vi "Inject.vi"(8 "error in (no error)":errorcluster, 9 "Injection Data":variant, 10 "Internal Message Queue":refnum<queue>, 11 "InteractionProcessor in":refnum<class "InteractionProcessor.lvclass">) -> (0 "error out":errorcluster, 3 "InteractionProcessor out":refnum<class "InteractionProcessor.lvclass">)   [LabVIEW 2023, in "HAF.lvlib" / "InteractionProcessor.lvclass"]
doc: "Add the Command Directors passed in the Message Data to the current set of Command Directors for processing."
uses:
  InteractionProcessor.lvclass
  Message.ctl
  All Internal Message Ids.ctl
  CommandDirector/CommandDirector.lvclass
  HAF.lvlib
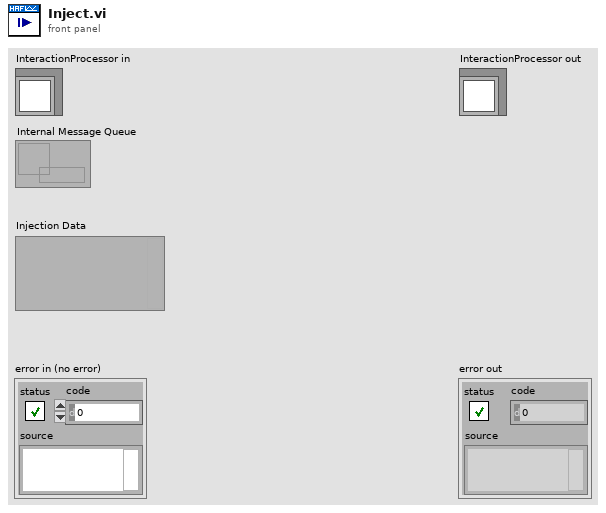
[diagram p1: front panel]
types:
  T1 = typedef "HAF.lvlib/All Internal Message Ids.ctl" = cluster{"Initialise":string, "Process":string, "Continue":string, "Done":string, "Pause":string, "Resume":string, "Stop":string, "Exit":string, "Inject":string}
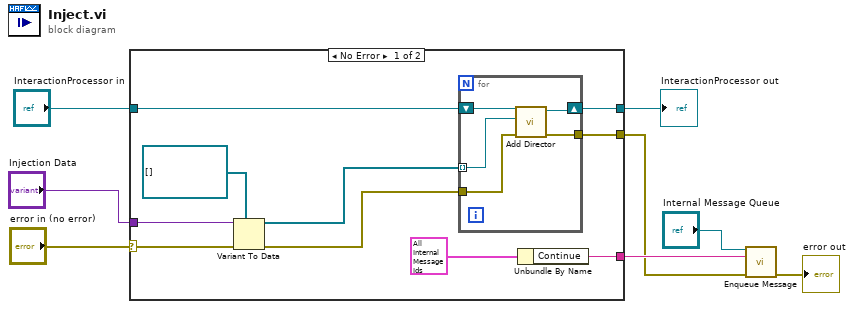
[diagram p0: block diagram]
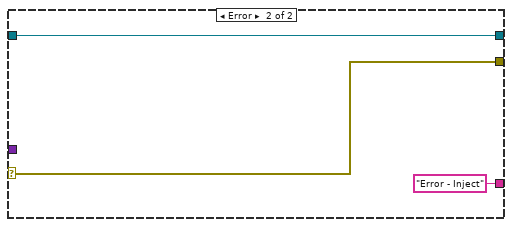
[diagram p2: hidden frame]
diagram:
  n1 = case shown="No Error" "error in (no error)" {
    selector: "error in (no error)" -> [w17 w26]
    tunnel: [w11 w26] -> w2
    tunnel: [w14 w25] -> w6
    tunnel: "InteractionProcessor in" -> [w16 w25]
    tunnel: "Injection Data" -> [w18 _]
    tunnel: [w12 "Error - Inject" ("Continue")] -> w3
    frame No Error {
      n2 = Variant To Data(error in=w17, type=refnum<class "CommandDirector.lvclass">[] [], Variant=w18) -> (data=w9:refnum<class "CommandDirector.lvclass">[], error out=w15:errorcluster)
      n3 = for {
        tunnel: w9 -> [w22] mode=indexing
        tunnel: w15 -> [w21]
        shift-right: [w20] -> w14
        shift-left: w16 -> [w23]
        tunnel: [w19] -> w11
        n4 = call-dynamic "Add Director.vi"("error in (no error)"=w21, "Command Director"=w22, "InteractionProcessor in"=w23) -> ("error out"=w19:errorcluster, "InteractionProcessor out"=w20:refnum<class "InteractionProcessor.lvclass">)  [unwired: 7 in]
      }
      n5 = Unbundle By Name(T1 {"Initialise"="Initialise", "Process"="Process", "Continue"="Continue", "Done"="Done", "Pause"="Pause", "Resume"="Resume", "Stop"="Stop", "Exit"="Exit", "Inject"=""} ("Message Ids")) -> ("Continue"=w12:string)
    }
    frame Error {
    }
  }
  "InteractionProcessor out" <- w6
  n6 = call "Enqueue Message.vi"("Message Queue In"="Internal Message Queue", "Message Id"=w3, "error in (no error)"=w2) -> ("error out"=→"error out":errorcluster)  [unwired: 11 in, 1 out]
